vi "timeAccessFormat (SubVI).vi"(1 "First Date":timestamp) -> (0 "result string":string)   [LabVIEW 2012]
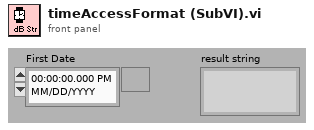
[diagram p1: front panel]
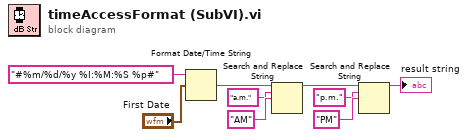
[diagram p0: block diagram]
diagram:
  n1 = Format Date/Time String(time format string (%c)="#%m/%d/%y %I:%M:%S %p#", seconds (now)="First Date") -> (date/time string=w5:string)  [unwired: 1 out]
  n2 = Search and Replace String(input string=w5, search string="a.m.", replace string="AM" ("replace string (\"\")")) -> (result string=w8:string)  [unwired: 1 in, 7 out]
  n3 = Search and Replace String(input string=w8, search string="p.m.", replace string="PM" ("replace string (\"\")")) -> (result string=→"result string":string)  [unwired: 1 in, 7 out]
